vi "DAQ - 24V.vi"(8 "error in":errorcluster, 11 "task in":refnum<k21>="MyDigitalInTask") -> (0 "error out":errorcluster, 2 "24V?":bool, 3 "task out":refnum<k21>)   [LabVIEW 2024]
doc: "Looking for voltage on this line using a 6525 DAQ. \nIf there is no 24V the loop will time out at 10 seconds.\nLink to start / end channel Vis."
uses:
  <vilib>/DAQmx/read.llb/DAQmx Read (Digital 1D Bool 1Chan 1Samp).vi
panel:
  out "Elapsed Time":dbl=1653.7379999160767
  out "DAQ Read 1":bool[](array[boolean])
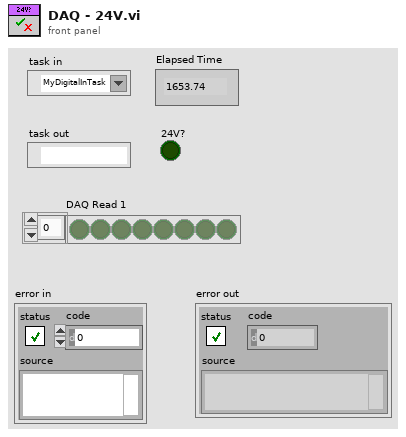
[diagram p1: front panel]
types:
  T1 = enum16{"Start Timer", "Get Time", "Pause", "Unpause"}
  T2 = cluster{"[0]":bool, "[1]":bool, "[2]":bool, "[3]":bool, "[4]":bool, "[5]":bool, "[6]":bool, "[7]":bool, "[8]":bool}
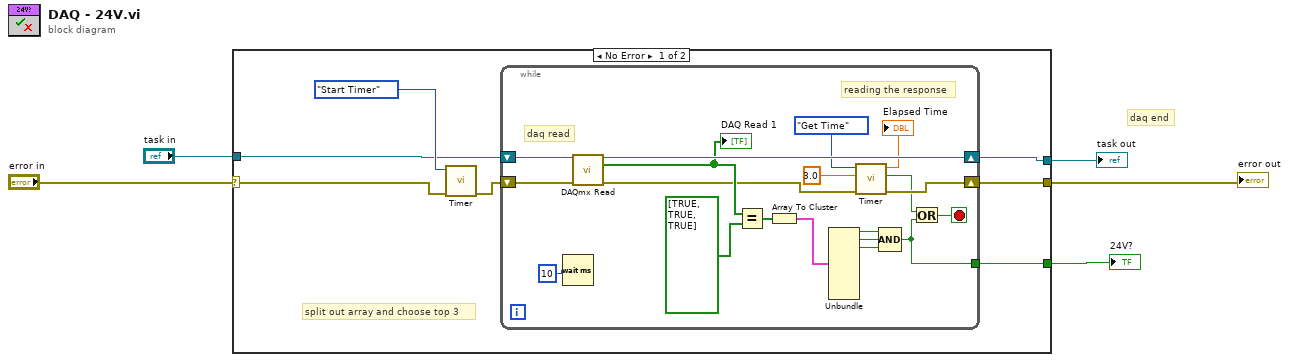
[diagram p0: block diagram]
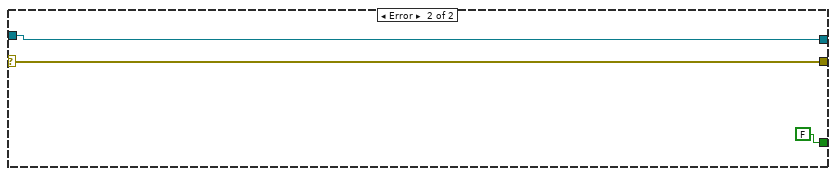
[diagram p2: hidden frame]
diagram:
  # "daq end"
  n1 = case shown="No Error" "error in" {
    selector: "error in" -> [w9 w33]
    tunnel: [w12 FALSE] -> w5
    tunnel: "task in" -> [w8 w34]
    tunnel: [w7 w34] -> w2
    tunnel: [w6 w33] -> w1
    frame No Error {
      # "split out array and choose top 3"
      n2 = call "Timer.vi"("error in (no error)"=w9, "Enum"=T1."Start Timer") -> ("error out"=w10:errorcluster)  [unwired: 6 in, 3 out]
      n3 = while {
        shift-right: [w30] -> w7
        shift-left: w8 -> [w31]
        shift-right: [w19] -> w6
        shift-left: w10 -> [w29]
        tunnel: [w18] -> w12
        stop <- w23 stop-if-true
        # "reading the response"
        # "daq read"
        n4 = Wait (ms)(milliseconds to wait=u32 10) -> ()  [unwired: 1 out]
        n5 = call-poly <vilib>:"DAQmx Read.vi"("task/channels in"=w31, "error in"=w29) -> ("task out"=w30:refnum<k21>, "data"=w25:bool[], "error out"=w20:errorcluster)  [unwired: 11 in]
        "DAQ Read 1" <- w25
        n6 = Equal?(x=w25, y=bool[] [TRUE, TRUE, TRUE] ("x")) -> (x = y?=w27:bool[])
        n7 = Array To Cluster(array=w27) -> (cluster=w26:T2)
        n8 = Unbundle(w26) -> ("[0]"=w24:bool, "[1]"=w15:bool, "[2]"=w13:bool)  [unwired: 6 out]
        n9 = call "Timer.vi"("error in (no error)"=w20, "Target Time"=3.0, "Enum"=T1."Get Time") -> ("error out"=w19:errorcluster, "Time Elapsed?"=w17:bool, "Elapsed Time"=→"Elapsed Time":dbl)  [unwired: 5 in, 1 out]
        n10 = Compound Arithmetic op=AND(w24, w15, w13) -> (w18:bool)
        n11 = Or(x=w17, y=w18) -> (x .or. y?=w23:bool)
      }
    }
    frame Error {
    }
  }
  "24V?" <- w5
  "error out" <- w1
  "task out" <- w2
